vi "Labspec GetMotorPosition.vi"(6 "Label Option":T1 items=[""=0, "Index to Value"=10, "Index to String"=20, "Full Index to Value"=30, "Full Index to String"=40], 8 "error in":errorcluster, 9 "Motor Name":T3, 10 "Mode":T2 items=["Value", "Step", "Index", "Size", "Full Size"], 11 "Automation Refnum In":refnum<k7>) -> (0 "error out":errorcluster, 2 "Position":variant, 3 "Automation Refnum Out":refnum<k7>)   [LabVIEW 2014]
uses:
  MoveMotor Motor Name.ctl
  GetMotorPosition Mode.ctl
  GetMotorPosition Label Option.ctl
panel:
  # "LICENSED MATERIALS – PROPERTY OF IBM\nCopyright IBM Corp. 2016,\nALL RIGHTS RESERVED"
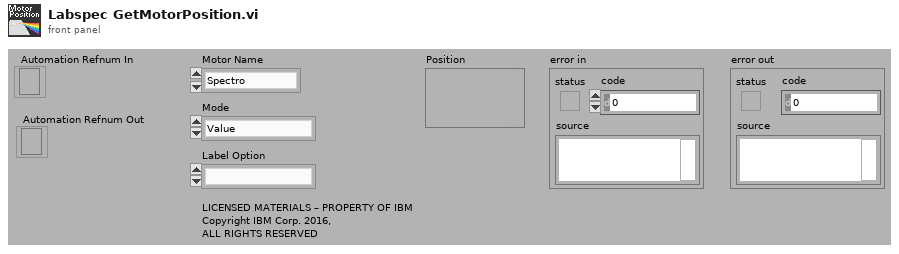
[diagram p1: front panel]
types:
  T1 = typedef "GetMotorPosition Label Option.ctl" = u16
  T2 = typedef "GetMotorPosition Mode.ctl" = u16
  T3 = typedef "MoveMotor Motor Name.ctl" = enum16{"Spectro", "Premono", "Grating", "Slit", "Hole", "X", "Y", "XT", "YT", "XL", "YL", "Z", "Laser", "Filter", "Objective", "Detector", "Detector Temperature"}
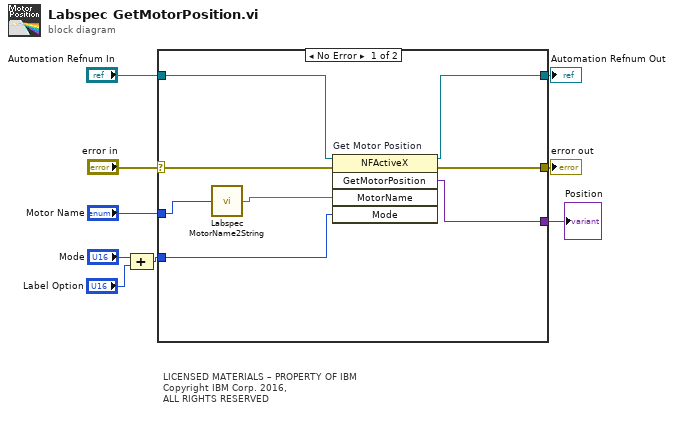
[diagram p0: block diagram]
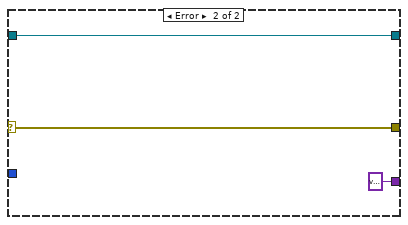
[diagram p2: hidden frame]
diagram:
  # "LICENSED MATERIALS – PROPERTY OF IBM\nCopyright IBM Corp. 2016,\nALL RIGHTS RESERVED"
  n1 = Compound Arithmetic op=ADD("Mode", "Label Option") -> (w2:T2)
  n2 = case shown="No Error" "error in" {
    selector: "error in" -> [w14 w19]
    tunnel: "Motor Name" -> [w13 _]
    tunnel: "Automation Refnum In" -> [w17 w20]
    tunnel: [w16 w20] -> w7
    tunnel: [w11 w19] -> w6
    tunnel: w2 -> [w15 _]
    tunnel: [w10 variant ("GetMotorPosition")] -> w3
    frame No Error {
      n3 = call "Labspec MotorName2String.vi"("Motor Name"=w13) -> ("PositionName"=w12:string)
      n4 = invoke on="Get Motor Position" class="NFActiveX" method="GetMotorPosition"(reference=w17, error in=w14, "MotorName"=w12, "Mode"=w15) -> (reference out=w16:refnum<k7>, error out=w11:errorcluster, "GetMotorPosition"=w10:variant)  [unwired: 1 in, 2 out]
    }
    frame Error {
    }
  }
  "error out" <- w6
  "Automation Refnum Out" <- w7
  "Position" <- w3
